vi "Initialize.vi"(8 "error in (no error)":errorcluster, 11 "ClassIn":refnum<class "NiPxi6733.lvclass">) -> (0 "error out":errorcluster, 3 "ClassOut":refnum<class "NiPxi6733.lvclass">)   [LabVIEW 2014, in "FGenPlugins.lvlib" / "NiPxi6733.lvclass"]
uses:
  NiPxi6733.lvclass
  <vilib>/DAQmx/create/channels.llb/DAQmx Create Channel (AO-Voltage-Basic).vi
  <resource>/objmgr/daqmx.rc
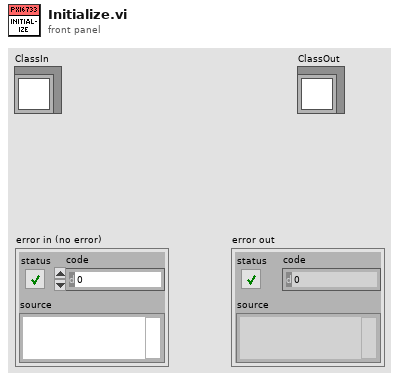
[diagram p1: front panel]
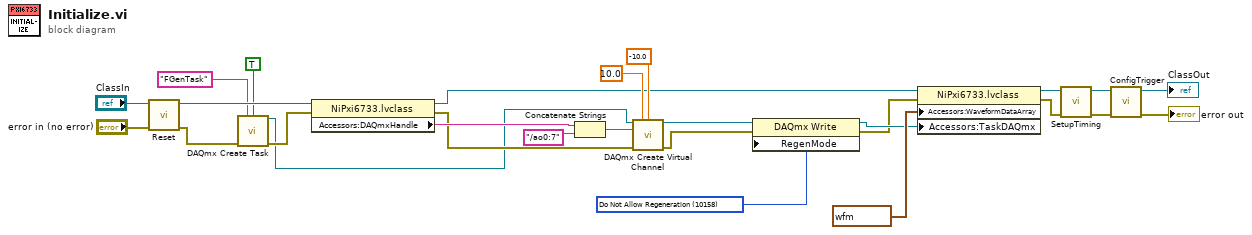
[diagram p0: block diagram]
diagram:
  w8 = 10158 items=["Allow Regeneration"=10097, "Do Not Allow Regeneration"=10158] ("RegenMode")
  n1 = call-dynamic "Reset.vi"("error in (no error)"="error in (no error)", "ClassIn"="ClassIn") -> ("error out"=w12:errorcluster, "ClassOut"=w18:refnum<class "NiPxi6733.lvclass">)  [unwired: 8 in]
  n2 = call <vilib>:"DAQmx Create Task.vi"("new task name"="FGenTask", "auto cleanup"=TRUE, "error in"=w12) -> ("task out"=w1:refnum<k21>, "error out"=w11:errorcluster)  [unwired: 11 in]
  n3 = property class="NiPxi6733.lvclass"(reference=w18, error in=w11) -> (reference out=w19:refnum<class "NiPxi6733.lvclass">, error out=w6:errorcluster, "Accessors:DAQmxHandle"=w7:tag)
  n4 = Concatenate Strings(w7, "/ao0:7" ("regular expression")) -> (w20:string)
  n5 = call-poly <vilib>:"DAQmx Create Virtual Channel.vi"("task in"=w1, "maximum value"=10.0, "minimum value"=-10.0, "physical channels"=w20, "error in"=w6) -> ("task out"=w5:refnum<k21>, "error out"=w4:errorcluster)  [unwired: 9 in]
  n6 = property class="DAQmx Write"(reference=w5, error in=w4, "RegenMode"=w8) -> (reference out=w3:refnum<k21>, error out=w2:errorcluster)
  n7 = property class="NiPxi6733.lvclass"(reference=w19, error in=w2, "Accessors:WaveformDataArray"=waveform(dbl)[] [{"t0"=timestamp(0 s since 1904-01-01), "dt"=1.0, "Y"=[0.0, 0.0, 0.0, 0.0, 0.0, 0.0, 0.0, 0.0, 0.0]}, {"t0"=timestamp(0 s since 1904-01-01), "dt"=1.0, "Y"=[0.0, 0.0, 0.0, 0.0, 0.0, 0.0, 0.0, 0.0, 0.0]}, {"t0"=timestamp(0 s since 1904-01-01), "dt"=1.0, "Y"=[0.0, 0.0, 0.0, 0.0, 0.0, 0.0, 0.0, 0.0, 0.0]}, {"t0"=timestamp(0 s since 1904-01-01), "dt"=1.0, "Y"=[0.0, 0.0, 0.0, 0.0, 0.0, 0.0, 0.0, 0.0, 0.0]}, {"t0"=timestamp(0 s since 1904-01-01), "dt"=1.0, "Y"=[0.0, 0.0, 0.0, 0.0, 0.0, 0.0, 0.0, 0.0, 0.0]}, {"t0"=timestamp(0 s since 1904-01-01), "dt"=1.0, "Y"=[0.0, 0.0, 0.0, 0.0, 0.0, 0.0, 0.0, 0.0, 0.0]}, {"t0"=timestamp(0 s since 1904-01-01), "dt"=1.0, "Y"=[0.0, 0.0, 0.0, 0.0, 0.0, 0.0, 0.0, 0.0, 0.0]}, {"t0"=timestamp(0 s since 1904-01-01), "dt"=1.0, "Y"=[0.0, 0.0, 0.0, 0.0, 0.0, 0.0, 0.0, 0.0, 0.0]}] ("WaveformDataArray"), "Accessors:TaskDAQmx"=w3) -> (reference out=w17:refnum<class "NiPxi6733.lvclass">, error out=w16:errorcluster)
  n8 = call "SetupTiming.vi"("error in (no error)"=w16, "ClassIn"=w17) -> ("error out"=w13:errorcluster, "ClassOut"=w14:refnum<class "NiPxi6733.lvclass">)  [unwired: 8 in]
  n9 = call-dynamic "ConfigTrigger.vi"("error in (no error)"=w13, "ClassIn"=w14) -> ("error out"=→"error out":errorcluster, "ClassOut"=→"ClassOut":refnum<class "NiPxi6733.lvclass">)  [unwired: 8 in]
